vi "SVL Integration (frequency).vi"   [LabVIEW 2017, in "SoundVib_Integration.lvlib"]
doc: "Converts acceleration to velocity or displacement using a frequency spectrum as the input. Wire data to the <B>spectrum</B> input to determine the polymorphic instance to use or manually select the instance."
uses:
  <vilib>/addons/Sound and Vibration/svt_Integration/SoundVib_Integration.lvlib
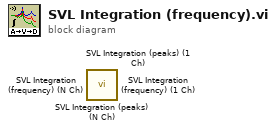
[diagram p0: block diagram]
diagram:
  n1 = call <vilib>:"SVL Integration (peaks) (N Ch).vi"() -> ()  [unwired: 16 in, 4 out]
  n2 = call <vilib>:"SVL Integration (peaks) (1 Ch).vi"() -> ()  [unwired: 16 in, 4 out]
  n3 = call <vilib>:"SVL Integration (frequency) (N Ch).vi"() -> ()  [unwired: 16 in, 4 out]
  n4 = call <vilib>:"SVL Integration (frequency) (1 Ch).vi"() -> ()  [unwired: 16 in, 4 out]
